vi "Timer Global Function Variable.vi"(8 "error in (no error)":errorcluster, 11 "Enum":enum16{"Init", "Read", "Set"}(ring)) -> (0 "error out":errorcluster, 2 "Timer Counting":bool, 3 "Time Elapsed":dbl)   [LabVIEW 2015]
panel:
  # "input"
  # "Output"
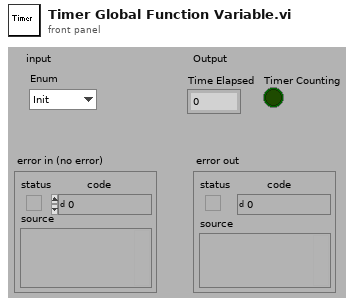
[diagram p1: front panel]
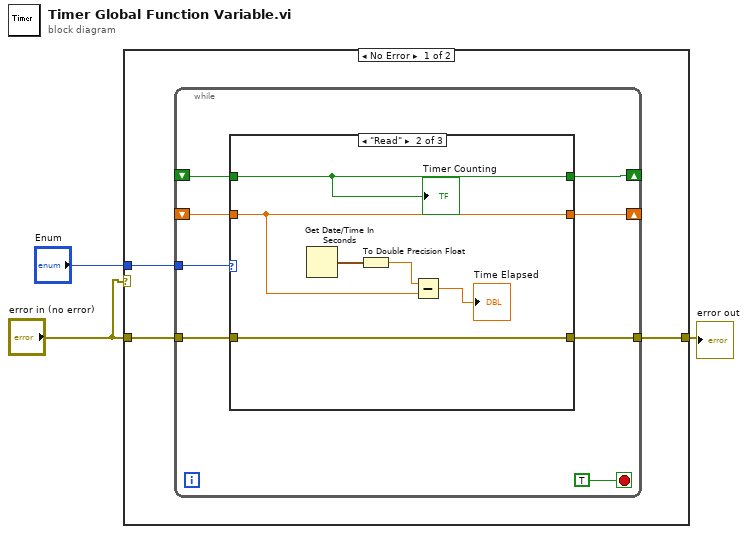
[diagram p0: block diagram]
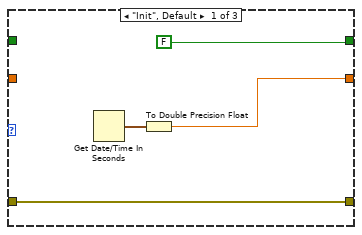
[diagram p2: hidden frame]
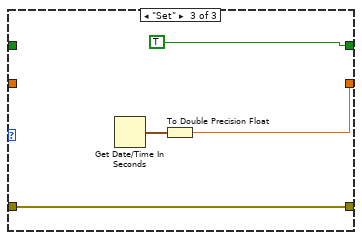
[diagram p3: hidden frame]
diagram:
  n1 = case shown="No Error" "error in (no error)" {
    tunnel: "Enum" -> [w6 _]
    tunnel: [w5 w29] -> w2
    tunnel: "error in (no error)" -> [w4 w29]
    frame No Error {
      n2 = while {
        shift-right: [w12] -> _
        shift-left: _ -> [w11]
        tunnel: w6 -> [w13]
        tunnel: [w10] -> w5
        tunnel: w4 -> [w9]
        shift-right: [w8] -> _
        shift-left: _ -> [w7]
        stop <- TRUE stop-if-true
        n3 = case shown="\"Read\"" w13 {
          tunnel: [w17 w20 w27] -> w12
          tunnel: w11 -> [_ w20 _]
          tunnel: [w16 w21 w26] -> w10
          tunnel: w9 -> [w16 w21 w26]
          tunnel: [FALSE w19 TRUE] -> w8
          tunnel: w7 -> [_ w19 _]
          frame "Init", Default {
            n4 = Get Date/Time In Seconds() -> (seconds since 1Jan1904=w18:timestamp)
            n5 = To Double Precision Float(number=w18) -> (double precision float=w17:dbl)
          }
          frame "Read" {
            n6 = Get Date/Time In Seconds() -> (seconds since 1Jan1904=w24:timestamp)
            n7 = To Double Precision Float(number=w24) -> (double precision float=w23:dbl)
            n8 = Subtract(x=w23, y=w20) -> (x-y=→"Time Elapsed":dbl)
            "Timer Counting" <- w19
          }
          frame "Set" {
            n9 = Get Date/Time In Seconds() -> (seconds since 1Jan1904=w28:timestamp)
            n10 = To Double Precision Float(number=w28) -> (double precision float=w27:dbl)
          }
        }
      }
    }
    frame Error {
    }
  }
  "error out" <- w2
